vi "draw_background.vi"(11 "input":picture) -> (3 "background":picture)   [LabVIEW 2025]
uses:
  <vilib>/Utility/miscctls.llb/LVBoundsTypeDef.ctl
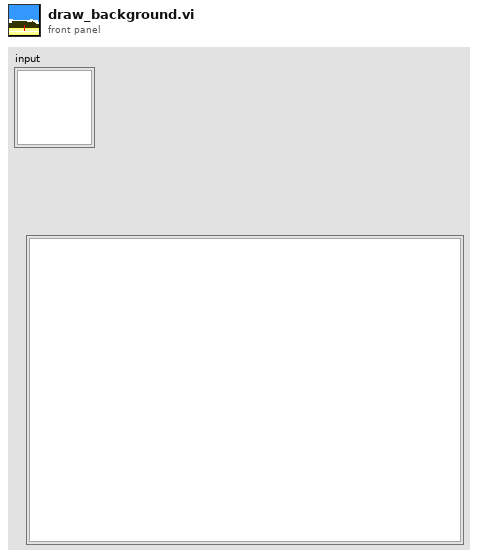
[diagram p1: front panel]
types:
  T1 = typedef "LVBoundsTypeDef.ctl" = cluster{"Width":u32, "Height":u32}
  T2 = typedef "imagedata.ctl" = cluster{"image type":i32, "image depth":i32, "image":u8[], "mask":u8[], "colors":u32[], "Rectangle":cluster{"left":i16, "top":i16, "right":i16, "bottom":i16}}
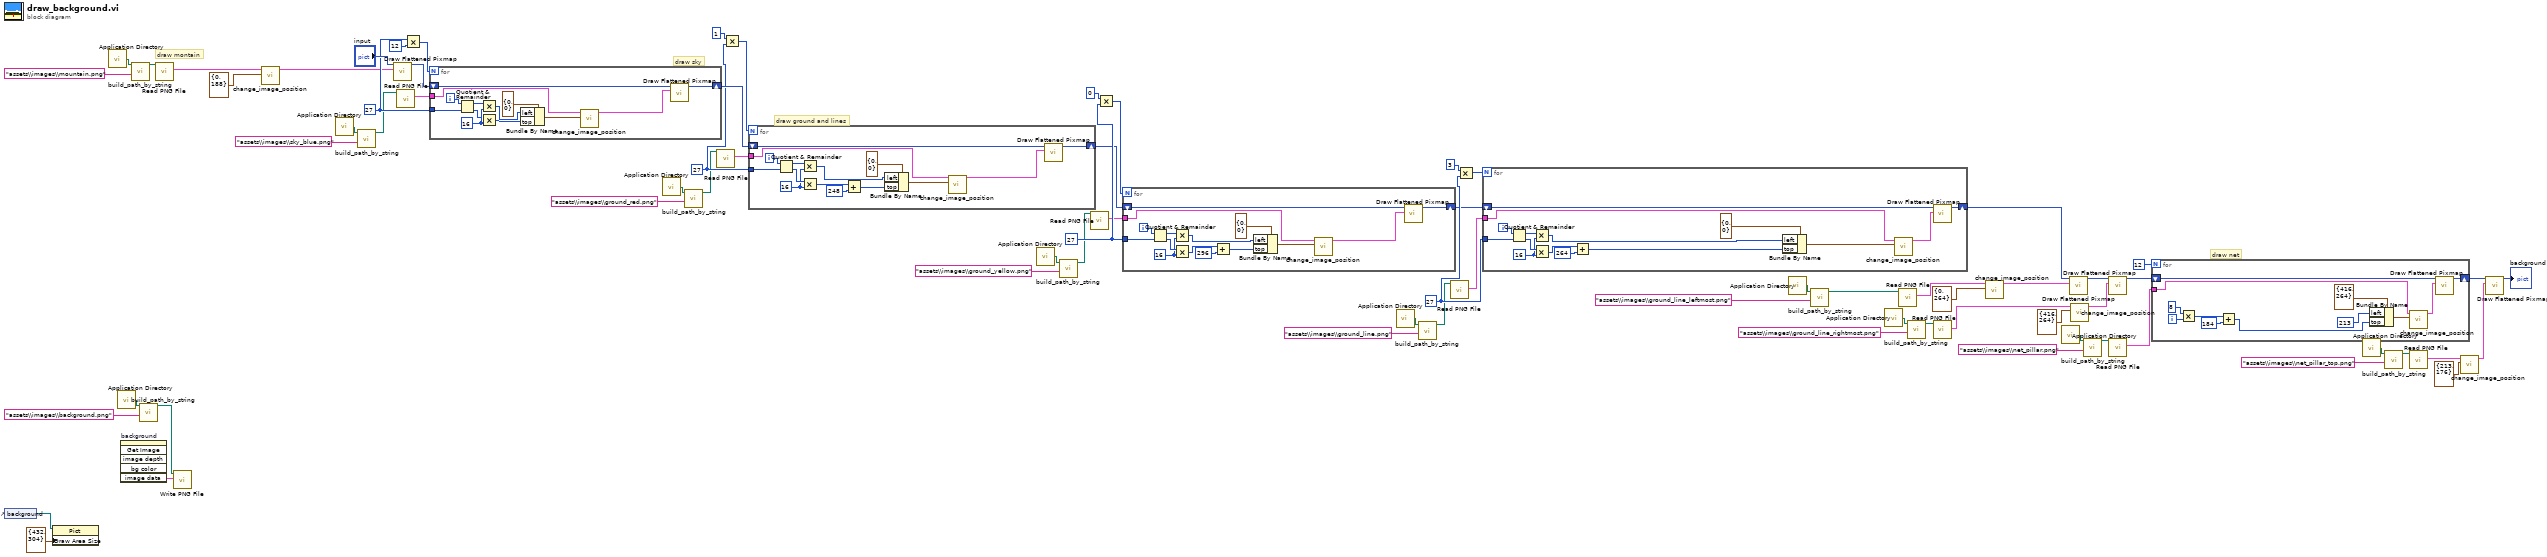
[diagram p0: block diagram]
diagram:
  w49 = 27
  w57 = 27
  w59 = 27
  w65 = 27
  # "draw net"
  # "draw ground and lines"
  # "draw sky"
  # "draw montain"
  n1 = control-ref of="background"() -> (w71:refnum<vi>)
  n2 = property on="Property Node" class="Pict"(reference=w71, "Draw Area Size"=T1 {"Width"=432, "Height"=304}) -> ()  [unwired: 1 in, 2 out]
  n3 = call <vilib>:"Application Directory.vi"() -> ("Application Directory"=w3:path)
  n4 = call <vilib>:"Application Directory.vi"() -> ("Application Directory"=w29:path)
  n5 = invoke on="background" class="Pict" method="Get Image"() -> ("image data"=w31:T2)  [unwired: 6 in, 5 out]
  n6 = call "build_path_by_string.vi"("String"="assets\\images\\mountain.png", "base path"=w3) -> ("appended path"=w1:path)  [unwired: 9 in]
  n7 = call "build_path_by_string.vi"("String"="assets\\images\\background.png", "base path"=w29) -> ("appended path"=w30:path)  [unwired: 9 in]
  n8 = call <vilib>:"Read PNG File.vi"("path to PNG file"=w1) -> ("image data"=w70:T2)  [unwired: 8 in, 2 out]
  n9 = call <vilib>:"Write PNG File.vi"("image data"=w31, "path to PNG file"=w30) -> ()  [unwired: 8 in, 2 out]
  n10 = call "change_image_position.vi"("position"=cluster{"left":i32, "top":i32} {"left"=0, "top"=188}, "image data in"=w70) -> ("image data out"=w58:T2)  [unwired: 9 in]
  n11 = call <vilib>:"Application Directory.vi"() -> ("Application Directory"=w5:path)
  n12 = call "build_path_by_string.vi"("String"="assets\\images\\sky_blue.png", "base path"=w5) -> ("appended path"=w4:path)  [unwired: 9 in]
  n13 = call <vilib>:"Draw Flattened Pixmap.vi"("image data"=w58, "picture"="input") -> ("new picture"=w68:picture)  [unwired: 7 in]
  n14 = call <vilib>:"Read PNG File.vi"("path to PNG file"=w4) -> ("image data"=w64:T2)  [unwired: 8 in, 2 out]
  n15 = Multiply(x=w65, y=12) -> (x*y=w67:i32)
  n16 = for {
    N: w67 -> [_]
    shift-right: [w84] -> w62
    shift-left: w68 -> [w85]
    tunnel: w65 -> [w78]
    tunnel: w64 -> [w74]
    i -> [w77]
    w79 = 16
    n17 = Quotient & Remainder(x=w77, y=w78) -> (x-y*floor(x/y)=w76:i32, floor(x/y)=w75:i32)
    n18 = Multiply(x=w76, y=w79) -> (x*y=w81:i32)
    n19 = Multiply(x=w75, y=w79) -> (x*y=w80:i32)
    n20 = Bundle By Name(cluster=cluster{"left":i32, "top":i32} {"left"=0, "top"=0} ("position"), "left"=w81, "top"=w80) -> (w82:cluster{"left":i32, "top":i32})
    n21 = call "change_image_position.vi"("position"=w82, "image data in"=w74) -> ("image data out"=w86:T2)  [unwired: 9 in]
    n22 = call <vilib>:"Draw Flattened Pixmap.vi"("image data"=w86, "picture"=w85) -> ("new picture"=w84:picture)  [unwired: 7 in]
  }
  n23 = call <vilib>:"Application Directory.vi"() -> ("Application Directory"=w9:path)
  n24 = call "build_path_by_string.vi"("String"="assets\\images\\ground_red.png", "base path"=w9) -> ("appended path"=w7:path)  [unwired: 9 in]
  n25 = call <vilib>:"Read PNG File.vi"("path to PNG file"=w7) -> ("image data"=w63:T2)  [unwired: 8 in, 2 out]
  n26 = Multiply(x=1, y=w59) -> (x*y=w61:i32)
  n27 = for {
    N: w61 -> [_]
    shift-right: [w99] -> w53
    shift-left: w62 -> [w100]
    tunnel: w59 -> [w95]
    tunnel: w63 -> [w92]
    i -> [w94]
    w87 = 16
    n28 = Quotient & Remainder(x=w94, y=w95) -> (x-y*floor(x/y)=w93:i32, floor(x/y)=w88:i32)
    n29 = Multiply(x=w93, y=w87) -> (x*y=w96:i32)
    n30 = Multiply(x=w88, y=w87) -> (x*y=w89:i32)
    n31 = Add(x=w89, y=248 ("top")) -> (x+y=w90:i32)
    n32 = Bundle By Name(cluster=cluster{"left":i32, "top":i32} {"left"=0, "top"=0} ("position"), "left"=w96, "top"=w90) -> (w97:cluster{"left":i32, "top":i32})
    n33 = call "change_image_position.vi"("position"=w97, "image data in"=w92) -> ("image data out"=w101:T2)  [unwired: 9 in]
    n34 = call <vilib>:"Draw Flattened Pixmap.vi"("image data"=w101, "picture"=w100) -> ("new picture"=w99:picture)  [unwired: 7 in]
  }
  n35 = call <vilib>:"Application Directory.vi"() -> ("Application Directory"=w12:path)
  n36 = call "build_path_by_string.vi"("String"="assets\\images\\ground_yellow.png", "base path"=w12) -> ("appended path"=w11:path)  [unwired: 9 in]
  n37 = call <vilib>:"Read PNG File.vi"("path to PNG file"=w11) -> ("image data"=w54:T2)  [unwired: 8 in, 2 out]
  n38 = Multiply(x=0, y=w57) -> (x*y=w55:i32)
  n39 = for {
    N: w55 -> [_]
    shift-right: [w114] -> w48
    shift-left: w53 -> [w115]
    tunnel: w57 -> [w110]
    tunnel: w54 -> [w107]
    i -> [w109]
    w102 = 16
    n40 = Quotient & Remainder(x=w109, y=w110) -> (x-y*floor(x/y)=w108:i32, floor(x/y)=w103:i32)
    n41 = Multiply(x=w108, y=w102) -> (x*y=w111:i32)
    n42 = Multiply(x=w103, y=w102) -> (x*y=w104:i32)
    n43 = Add(x=w104, y=296 ("top")) -> (x+y=w105:i32)
    n44 = Bundle By Name(cluster=cluster{"left":i32, "top":i32} {"left"=0, "top"=0} ("position"), "left"=w111, "top"=w105) -> (w112:cluster{"left":i32, "top":i32})
    n45 = call "change_image_position.vi"("position"=w112, "image data in"=w107) -> ("image data out"=w116:T2)  [unwired: 9 in]
    n46 = call <vilib>:"Draw Flattened Pixmap.vi"("image data"=w116, "picture"=w115) -> ("new picture"=w114:picture)  [unwired: 7 in]
  }
  n47 = call <vilib>:"Application Directory.vi"() -> ("Application Directory"=w15:path)
  n48 = call "build_path_by_string.vi"("String"="assets\\images\\ground_line.png", "base path"=w15) -> ("appended path"=w14:path)  [unwired: 9 in]
  n49 = call <vilib>:"Read PNG File.vi"("path to PNG file"=w14) -> ("image data"=w52:T2)  [unwired: 8 in, 2 out]
  n50 = Multiply(x=3, y=w49) -> (x*y=w51:i32)
  n51 = for {
    N: w51 -> [_]
    shift-right: [w129] -> w41
    shift-left: w48 -> [w130]
    tunnel: w49 -> [w125]
    tunnel: w52 -> [w122]
    i -> [w124]
    w117 = 16
    n52 = Quotient & Remainder(x=w124, y=w125) -> (x-y*floor(x/y)=w123:i32, floor(x/y)=w118:i32)
    n53 = Multiply(x=w123, y=w117) -> (x*y=w126:i32)
    n54 = Multiply(x=w118, y=w117) -> (x*y=w119:i32)
    n55 = Add(x=w119, y=264 ("top")) -> (x+y=w120:i32)
    n56 = Bundle By Name(cluster=cluster{"left":i32, "top":i32} {"left"=0, "top"=0} ("position"), "left"=w126, "top"=w120) -> (w127:cluster{"left":i32, "top":i32})
    n57 = call "change_image_position.vi"("position"=w127, "image data in"=w122) -> ("image data out"=w131:T2)  [unwired: 9 in]
    n58 = call <vilib>:"Draw Flattened Pixmap.vi"("image data"=w131, "picture"=w130) -> ("new picture"=w129:picture)  [unwired: 7 in]
  }
  n59 = call <vilib>:"Application Directory.vi"() -> ("Application Directory"=w18:path)
  n60 = call "build_path_by_string.vi"("String"="assets\\images\\ground_line_leftmost.png", "base path"=w18) -> ("appended path"=w17:path)  [unwired: 9 in]
  n61 = call <vilib>:"Application Directory.vi"() -> ("Application Directory"=w21:path)
  n62 = call <vilib>:"Read PNG File.vi"("path to PNG file"=w17) -> ("image data"=w47:T2)  [unwired: 8 in, 2 out]
  n63 = call "build_path_by_string.vi"("String"="assets\\images\\ground_line_rightmost.png", "base path"=w21) -> ("appended path"=w19:path)  [unwired: 9 in]
  n64 = call <vilib>:"Read PNG File.vi"("path to PNG file"=w19) -> ("image data"=w46:T2)  [unwired: 8 in, 2 out]
  n65 = call "change_image_position.vi"("position"=cluster{"left":i32, "top":i32} {"left"=0, "top"=264}, "image data in"=w47) -> ("image data out"=w43:T2)  [unwired: 9 in]
  n66 = call <vilib>:"Application Directory.vi"() -> ("Application Directory"=w24:path)
  n67 = call <vilib>:"Draw Flattened Pixmap.vi"("image data"=w43, "picture"=w41) -> ("new picture"=w40:picture)  [unwired: 7 in]
  n68 = call "change_image_position.vi"("position"=cluster{"left":i32, "top":i32} {"left"=416, "top"=264}, "image data in"=w46) -> ("image data out"=w42:T2)  [unwired: 9 in]
  n69 = call "build_path_by_string.vi"("String"="assets\\images\\net_pillar.png", "base path"=w24) -> ("appended path"=w22:path)  [unwired: 9 in]
  n70 = call <vilib>:"Draw Flattened Pixmap.vi"("image data"=w42, "picture"=w40) -> ("new picture"=w37:picture)  [unwired: 7 in]
  n71 = call <vilib>:"Read PNG File.vi"("path to PNG file"=w22) -> ("image data"=w39:T2)  [unwired: 8 in, 2 out]
  n72 = for {
    N: 12 -> [_]
    shift-right: [w138] -> w33
    shift-left: w37 -> [w139]
    tunnel: w39 -> [w143]
    i -> [w133]
    n73 = Multiply(x=8, y=w133) -> (x*y=w132:i32)
    n74 = Add(x=w132, y=184) -> (x+y=w136:i32)
    n75 = Bundle By Name(cluster=cluster{"left":i32, "top":i32} {"left"=416, "top"=264} ("position"), "left"=213, "top"=w136) -> (w141:cluster{"left":i32, "top":i32})
    n76 = call "change_image_position.vi"("position"=w141, "image data in"=w143) -> ("image data out"=w140:T2)  [unwired: 9 in]
    n77 = call <vilib>:"Draw Flattened Pixmap.vi"("image data"=w140, "picture"=w139) -> ("new picture"=w138:picture)  [unwired: 7 in]
  }
  n78 = call <vilib>:"Application Directory.vi"() -> ("Application Directory"=w27:path)
  n79 = call "build_path_by_string.vi"("String"="assets\\images\\net_pillar_top.png", "base path"=w27) -> ("appended path"=w26:path)  [unwired: 9 in]
  n80 = call <vilib>:"Read PNG File.vi"("path to PNG file"=w26) -> ("image data"=w36:T2)  [unwired: 8 in, 2 out]
  n81 = call "change_image_position.vi"("position"=cluster{"left":i32, "top":i32} {"left"=213, "top"=176}, "image data in"=w36) -> ("image data out"=w32:T2)  [unwired: 9 in]
  n82 = call <vilib>:"Draw Flattened Pixmap.vi"("image data"=w32, "picture"=w33) -> ("new picture"=→"background":picture)  [unwired: 7 in]
